vi "W7X1DPut.vi"(4 "dimensions":i64[](array[numeric])=[1428413878000000000, -1], 7 "Unit":string="s", 9 "values":T1(array[cluster]), 10 "SigJSONbuffer":string, 11 "SigLabel":string="MTau") -> (0 "Parlog error out":errorcluster, 1 "file path written":string, 2 "headers parms":string, 3 "body Parlog":string, 5 "body":string, 6 "headers":string)   [LabVIEW 2014]
uses:
  <vilib>/httpClient/POSTBuffer.vi
  <vilib>/httpClient/LabVIEWHTTPClient.lvlib
panel:
  out "JSON string":string
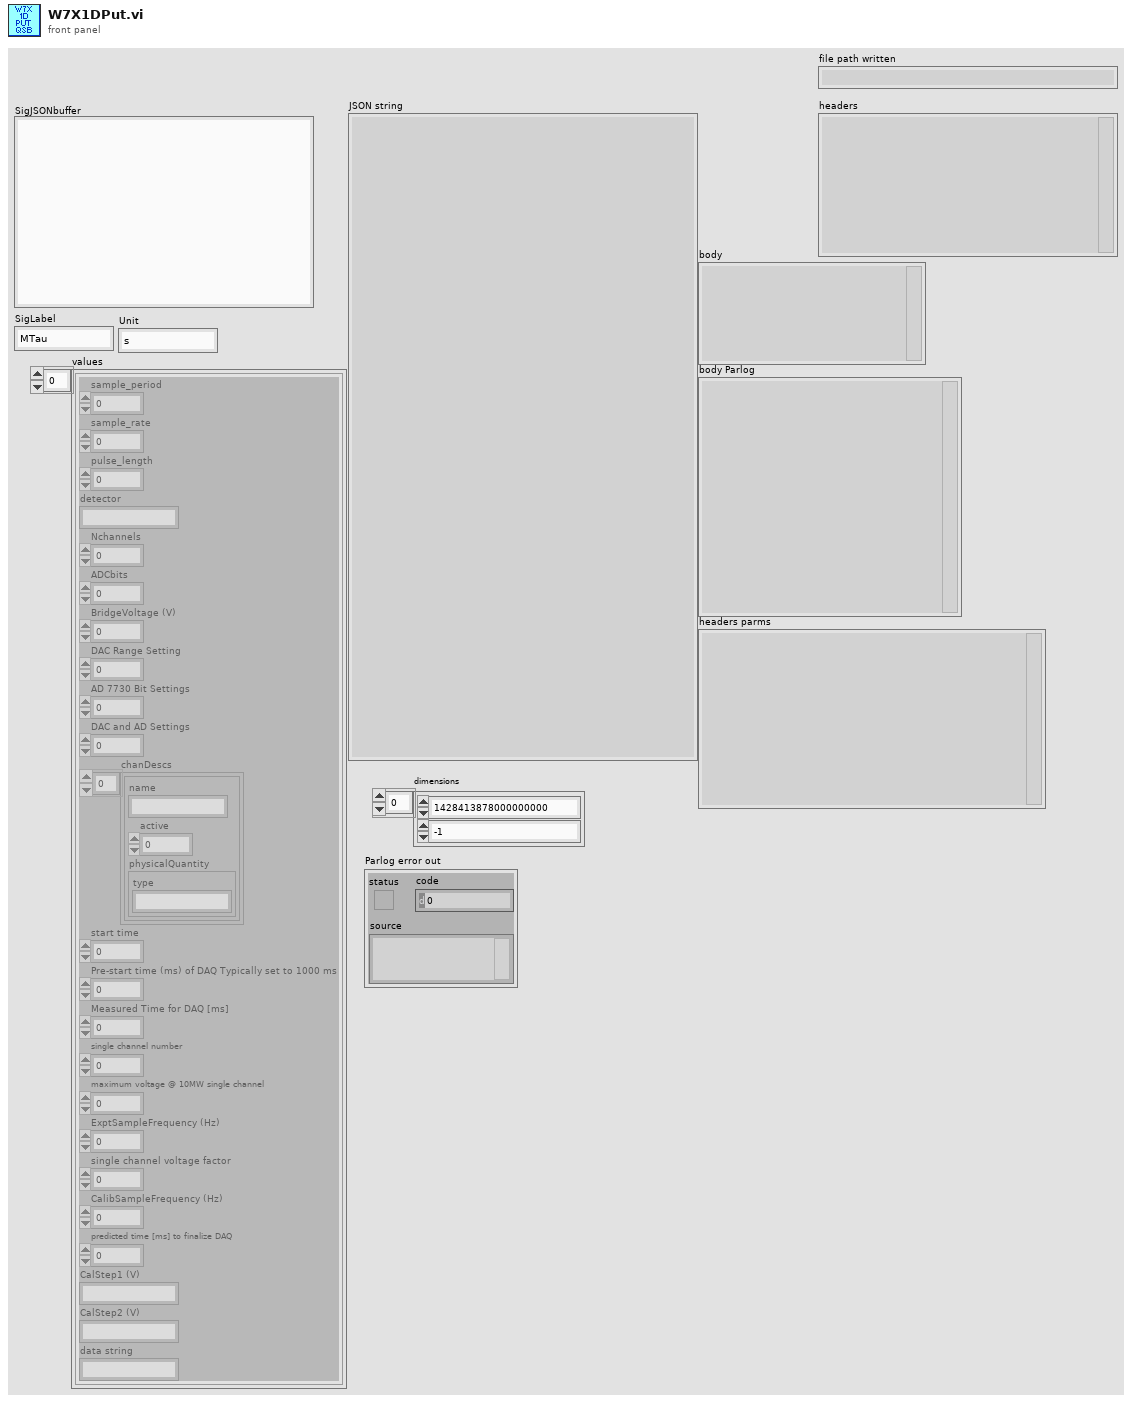
[diagram p1: front panel]
types:
  T1 = cluster{"sample_period":dbl, "sample_rate":dbl, "pulse_length":dbl, "detector":string, "Nchannels":i16, "ADCbits":i16, "BridgeVoltage (V)":sgl, "DAC Range Setting":u8, "AD 7730 Bit Settings":i32, "DAC and AD Settings":i32, "chanDescs":cluster{"name":string, "active":i32, "physicalQuantity":cluster{"type":string}}[], "start time":i64, "Pre-start time (ms) of DAQ Typically set to 1000 ms":i32, "Measured Time for DAQ [ms] ":u32, "single channel number":i64, "maximum voltage @ 10MW single channel":dbl, "ExptSampleFrequency (Hz)":sgl, "single channel voltage factor":dbl, "CalibSampleFrequency (Hz)":sgl, "predicted time [ms] to finalize DAQ":dbl, "CalStep1 (V)":string, "CalStep2 (V)":string, "data string":string}[]
  T2 = cluster{"sample_period":dbl, "sample_rate":dbl, "pulse_length":dbl, "detector":string, "Nchannels":i16, "ADCbits":i16, "BridgeVoltage (V)":sgl, "DAC Range Setting":u8, "AD 7730 Bit Settings":i32, "DAC and AD Settings":i32, "chanDescs":cluster{"name":string, "active":i32, "physicalQuantity":cluster{"type":string}}[], "start time":i64, "Pre-start time (ms) of DAQ Typically set to 1000 ms":i32, "Measured Time for DAQ [ms] ":u32, "single channel number":i64, "maximum voltage @ 10MW single channel":dbl, "ExptSampleFrequency (Hz)":sgl, "single channel voltage factor":dbl, "CalibSampleFrequency (Hz)":sgl, "predicted time [ms] to finalize DAQ":dbl, "CalStep1 (V)":string, "CalStep2 (V)":string, "data string":string}
  T3 = cluster{"name":string, "active":i32, "physicalQuantity":cluster{"type":string}}[]
  T4 = cluster{"name":string, "active":i32, "physicalQuantity":cluster{"type":string}}
  T5 = typedef "LabVIEWHTTPClient.lvlib/ClientHandle.ctl" = refnum<k1>
  T6 = cluster{"label":string, "values":cluster{"sample_period":dbl, "sample_rate":dbl, "pulse_length":dbl, "detector":string, "Nchannels":i16, "ADCbits":i16, "BridgeVoltage (V)":sgl, "DAC Range Setting":u8, "AD 7730 Bit Settings":i32, "DAC and AD Settings":i32, "chanDescs":cluster{"name":string, "active":i32, "physicalQuantity":cluster{"type":string}}[], "start time":i64, "Pre-start time (ms) of DAQ Typically set to 1000 ms":i32, "Measured Time for DAQ [ms] ":u32, "single channel number":i64, "maximum voltage @ 10MW single channel":dbl, "ExptSampleFrequency (Hz)":sgl, "single channel voltage factor":dbl, "CalibSampleFrequency (Hz)":sgl, "predicted time [ms] to finalize DAQ":dbl, "CalStep1 (V)":string, "CalStep2 (V)":string, "data string":string}[], "dimensions":i64[]}
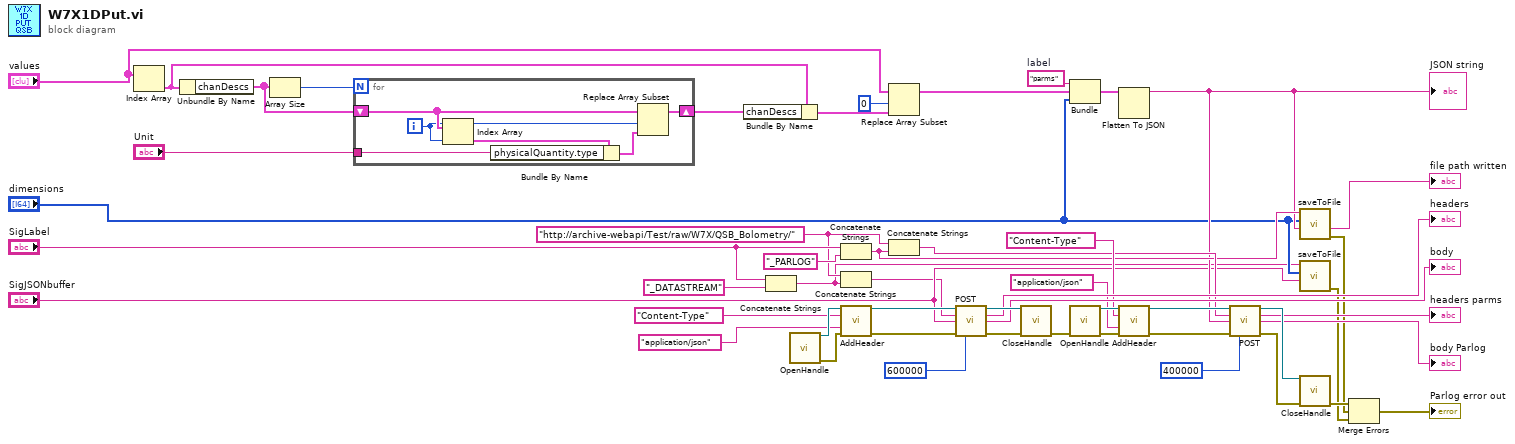
[diagram p0: block diagram]
diagram:
  w38 = "parms"  # label
  w13 = "http://archive-webapi/Test/raw/W7X/QSB_Bolometry/" ("url")
  n1 = Index Array(array="values") -> (element=w6:T2)  [unwired: 1 in]
  n2 = Unbundle By Name(w6) -> ("chanDescs"=w2:T3)
  n3 = Array Size(array=w2) -> (size(s)=w1:i32)
  n4 = for {
    N: w1 -> [_]
    tunnel: "Unit" -> [w56]
    shift-right: [w52] -> w3
    shift-left: w2 -> [w54]
    i -> [w51]
    n5 = Index Array(array=w54, index=w51) -> (element=w55:T4)
    n6 = Bundle By Name(cluster=w55, "physicalQuantity.type"=w56) -> (w53:T4)
    n7 = Replace Array Subset(array=w54, new element=w53, index=w51) -> (w52:T3)
  }
  n8 = Bundle By Name(cluster=w6, "chanDescs"=w3) -> (w5:T2)
  n9 = Concatenate Strings("SigLabel", "_DATASTREAM" ("string")) -> (w12:string)
  n10 = call <vilib>:"OpenHandle.vi"() -> ("client handle out"=w47:T5, "error out"=w46:errorcluster)  [unwired: 14 in]
  n11 = Concatenate Strings("SigLabel", "_PARLOG" ("replace string (\"\")")) -> (w18:string)
  n12 = Concatenate Strings(w13, w12) -> (w14:string)
  n13 = call <vilib>:"AddHeader.vi"("client handle"=w47, "header"="Content-Type", "value"="application/json", "error in (no error)"=w46) -> ("client handle out"=w45:T5, "error out"=w44:errorcluster)  [unwired: 10 in]
  n14 = Replace Array Subset(array="values", new element=w5, index=0) -> (w36:T1)
  n15 = Concatenate Strings(w13, w18) -> (w19:string)
  n16 = call-poly <vilib>:"POST.vi"("client handle"=w45, "url"=w14, "buffer"="SigJSONbuffer", "error in (no error)"=w44, "timeout (10000)"=600000) -> ("client handle out"=w50:T5, "headers"=→"headers":string, "body"=→"body":string, "error out"=w49:errorcluster)  [unwired: 7 in]
  n17 = call <vilib>:"CloseHandle.vi"("client handle"=w50, "error in (no error)"=w49) -> ("error out"=w11:errorcluster)  [unwired: 13 in]
  n18 = Bundle("label"=w38, "values"=w36, "dimensions"="dimensions") -> (w37:T6)  [unwired: 1 in]
  n19 = call <vilib>:"OpenHandle.vi"("error in (no error)"=w11) -> ("client handle out"=w32:T5, "error out"=w31:errorcluster)  [unwired: 13 in]
  n20 = Flatten To JSON(anything=w37) -> (JSON string=w17:string)  [unwired: 2 in, 1 out]
  "JSON string" <- w17
  n21 = call <vilib>:"AddHeader.vi"("client handle"=w32, "header"="Content-Type", "value"="application/json", "error in (no error)"=w31) -> ("client handle out"=w30:T5, "error out"=w29:errorcluster)  [unwired: 10 in]
  n22 = call-poly <vilib>:"POST.vi"("client handle"=w30, "url"=w19, "buffer"=w17, "error in (no error)"=w29, "timeout (10000)"=400000) -> ("client handle out"=w35:T5, "headers"=→"headers parms":string, "body"=→"body Parlog":string, "error out"=w34:errorcluster)  [unwired: 7 in]
  n23 = call "saveToFile.vi"("SigJSONbuffer"=w17, "dimensions"="dimensions", "String"=w18) -> ("error out"=w20:errorcluster, "resulting string"=→"file path written":string)  [unwired: 7 in]
  n24 = call "saveToFile.vi"("SigJSONbuffer"="SigJSONbuffer", "dimensions"="dimensions", "String"=w12) -> ("error out"=w10:errorcluster)  [unwired: 7 in, 1 out]
  n25 = call <vilib>:"CloseHandle.vi"("client handle"=w35, "error in (no error)"=w34) -> ("error out"=w24:errorcluster)  [unwired: 13 in]
  n26 = Merge Errors(w24, w20, w10) -> (→"Parlog error out":errorcluster)
